vi "数据处理直接插入整合 (子VI).vi"   [LabVIEW 2016, in "数据传输系统-05.lvlib"]
types:
  T1 = cluster{"PH":string[][], "CODCr":string[][], "氨氮":string[][], "CODMn":string[][], "总氮":string[][], "总磷":string[][], "电导率":string[][], "水温":string[][], "COD":string[][], "DO":string[][], "浊度":string[][], "叶绿素":string[][], "藻密度":string[][], "铜":string[][], "盐度":string[][], "水位":string[][], "流速":string[][], "方向":string[][], "瞬时流量":string[][], "累积流量":string[][], "正累积流量":string[][], "负累积流量":string[][], "亚硝酸盐":string[][], "硫化物":string[][], "ORP":string[][], "铅":string[][], "镉":string[][], "锌":string[][], "镍":string[][], "锰":string[][], "汞":string[][], "气温":string[][], "气压":string[][], "风速":string[][], "风向":string[][], "空气温度":string[][], "相对湿度":string[][], "分钟雨量":string[][], "小时雨量":string[][], "日雨量":string[][], "累积雨量":string[][], "盐度":string[][], "磷酸盐":string[][], "硝氮":string[][], "氟化物":string[][], "挥发酚":string[][], "氯化物":string[][], "蓝绿藻":string[][], "余氯":string[][], "综合生物毒性":string[][], "水深":string[][]}
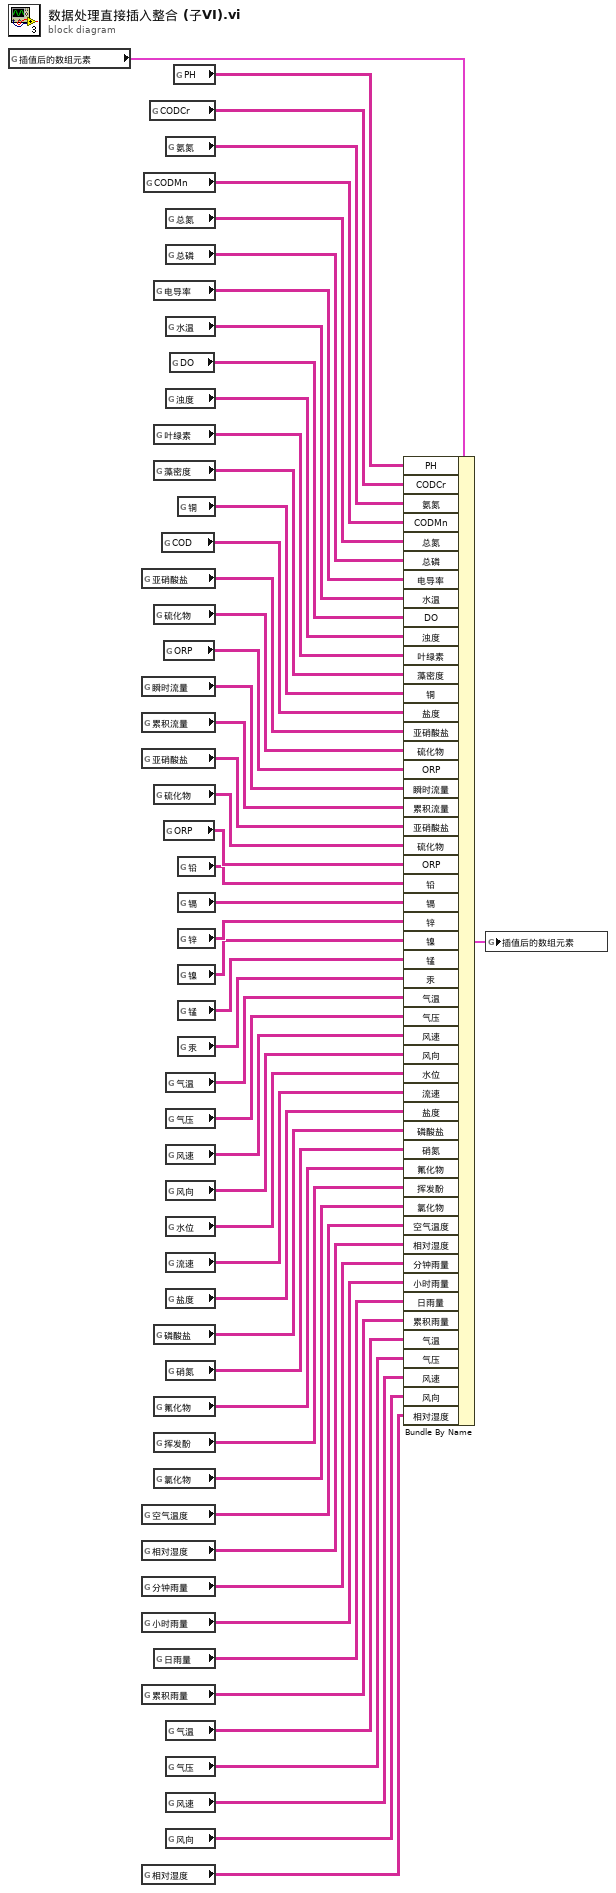
[diagram p0: block diagram]
diagram:
  n1 = global read "插值后的新数组.vi" "插值后的数组元素"() -> (w39:T1)
  n2 = global read "全局 所有参数.vi" "亚硝酸盐"() -> (w36:string[][])
  n3 = global read "全局 所有参数.vi" "瞬时流量"() -> (w34:string[][])
  n4 = global read "全局 所有参数.vi" "累积流量"() -> (w33:string[][])
  n5 = global read "全局 所有参数.vi" "亚硝酸盐"() -> (w32:string[][])
  n6 = global read "全局 所有参数.vi" "空气温度"() -> (w11:string[][])
  n7 = global read "全局 所有参数.vi" "相对湿度"() -> (w10:string[][])
  n8 = global read "全局 所有参数.vi" "分钟雨量"() -> (w9:string[][])
  n9 = global read "全局 所有参数.vi" "小时雨量"() -> (w8:string[][])
  n10 = global read "全局 所有参数.vi" "累积雨量"() -> (w6:string[][])
  n11 = global read "全局 所有参数.vi" "相对湿度"() -> (w1:string[][])
  n12 = global read "全局 所有参数.vi" "CODMn"() -> (w50:string[][])
  n13 = global read "全局 所有参数.vi" "CODCr"() -> (w52:string[][])
  n14 = global read "全局 所有参数.vi" "电导率"() -> (w47:string[][])
  n15 = global read "全局 所有参数.vi" "叶绿素"() -> (w43:string[][])
  n16 = global read "全局 所有参数.vi" "藻密度"() -> (w42:string[][])
  n17 = global read "全局 所有参数.vi" "硫化物"() -> (w37:string[][])
  n18 = global read "全局 所有参数.vi" "硫化物"() -> (w31:string[][])
  n19 = global read "全局 所有参数.vi" "磷酸盐"() -> (w16:string[][])
  n20 = global read "全局 所有参数.vi" "氟化物"() -> (w14:string[][])
  n21 = global read "全局 所有参数.vi" "挥发酚"() -> (w13:string[][])
  n22 = global read "全局 所有参数.vi" "氯化物"() -> (w12:string[][])
  n23 = global read "全局 所有参数.vi" "日雨量"() -> (w7:string[][])
  n24 = global read "全局 所有参数.vi" "COD"() -> (w40:string[][])
  n25 = global read "全局 所有参数.vi" "ORP"() -> (w38:string[][])
  n26 = global read "全局 所有参数.vi" "ORP"() -> (w30:string[][])
  n27 = global read "全局 所有参数.vi" "氨氮"() -> (w51:string[][])
  n28 = global read "全局 所有参数.vi" "总氮"() -> (w49:string[][])
  n29 = global read "全局 所有参数.vi" "总磷"() -> (w48:string[][])
  n30 = global read "全局 所有参数.vi" "水温"() -> (w46:string[][])
  n31 = global read "全局 所有参数.vi" "浊度"() -> (w44:string[][])
  n32 = global read "全局 所有参数.vi" "气温"() -> (w23:string[][])
  n33 = global read "全局 所有参数.vi" "气压"() -> (w22:string[][])
  n34 = global read "全局 所有参数.vi" "风速"() -> (w21:string[][])
  n35 = global read "全局 所有参数.vi" "风向"() -> (w20:string[][])
  n36 = global read "全局 所有参数.vi" "水位"() -> (w19:string[][])
  n37 = global read "全局 所有参数.vi" "流速"() -> (w18:string[][])
  n38 = global read "全局 所有参数.vi" "盐度"() -> (w17:string[][])
  n39 = global read "全局 所有参数.vi" "硝氮"() -> (w15:string[][])
  n40 = global read "全局 所有参数.vi" "气温"() -> (w5:string[][])
  n41 = global read "全局 所有参数.vi" "气压"() -> (w4:string[][])
  n42 = global read "全局 所有参数.vi" "风速"() -> (w3:string[][])
  n43 = global read "全局 所有参数.vi" "风向"() -> (w2:string[][])
  n44 = global read "全局 所有参数.vi" "DO"() -> (w45:string[][])
  n45 = global read "全局 所有参数.vi" "PH"() -> (w53:string[][])
  n46 = global read "全局 所有参数.vi" "铜"() -> (w41:string[][])
  n47 = global read "全局 所有参数.vi" "铅"() -> (w29:string[][])
  n48 = global read "全局 所有参数.vi" "镉"() -> (w28:string[][])
  n49 = global read "全局 所有参数.vi" "锌"() -> (w27:string[][])
  n50 = global read "全局 所有参数.vi" "镍"() -> (w26:string[][])
  n51 = global read "全局 所有参数.vi" "锰"() -> (w25:string[][])
  n52 = global read "全局 所有参数.vi" "汞"() -> (w24:string[][])
  n53 = Bundle By Name(cluster=w39, "PH"=w53, "CODCr"=w52, "氨氮"=w51, "CODMn"=w50, "总氮"=w49, "总磷"=w48, "电导率"=w47, "水温"=w46, "DO"=w45, "浊度"=w44, "叶绿素"=w43, "藻密度"=w42, "铜"=w41, "盐度"=w40, "亚硝酸盐"=w36, "硫化物"=w37, "ORP"=w38, "瞬时流量"=w34, "累积流量"=w33, "亚硝酸盐"=w32, "硫化物"=w31, "ORP"=w30, "铅"=w29, "镉"=w28, "锌"=w27, "镍"=w26, "锰"=w25, "汞"=w24, "气温"=w23, "气压"=w22, "风速"=w21, "风向"=w20, "水位"=w19, "流速"=w18, "盐度"=w17, "磷酸盐"=w16, "硝氮"=w15, "氟化物"=w14, "挥发酚"=w13, "氯化物"=w12, "空气温度"=w11, "相对湿度"=w10, "分钟雨量"=w9, "小时雨量"=w8, "日雨量"=w7, "累积雨量"=w6, "气温"=w5, "气压"=w4, "风速"=w3, "风向"=w2, "相对湿度"=w1) -> (w35:T1)
  n54 = global write "插值后的新数组.vi" "插值后的数组元素"(w35) -> ()
